vi "TankOverview.vi"() -> ()   [LabVIEW 2021]
uses:
  <vilib>/addons/control/pid/pid.llb/PID (DBL).vi
  <vilib>/addons/control/pid/NI_PID_pid.lvlib
panel:
  in  "Fout":dbl(slide) scale=0.0..10.0
  out "Tank":dbl(slide) scale=0.0..20.0
  out "Tank Level [cm]":dbl(graph)
  in  "PID gains":T1={"proportional gain (Kc)"=1.0, "integral time (Ti, min)"=0.01, "derivative time (Td, min)"=0.0} {"derivative time (Td, min)" format="%.3f"; "integral time (Ti, min)" format="%.3f"; "proportional gain (Kc)" format="%.3f"}
  in  "Hset":dbl(slide) scale=0.0..20.0
  in  "stop":bool
  in  "Ts [ms]":dbl
  in  "Tf [s]":dbl
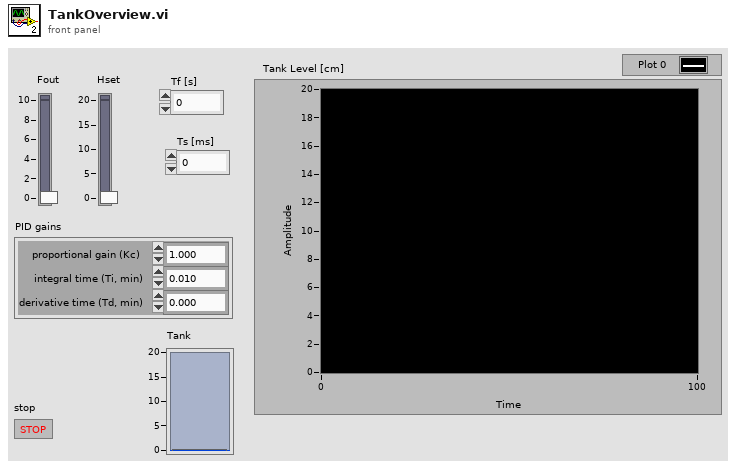
[diagram p1: front panel]
types:
  T1 = cluster{"proportional gain (Kc)":dbl, "integral time (Ti, min)":dbl, "derivative time (Td, min)":dbl}
  T2 = enum16{"Read", "Write", "ReadWrite", "BufferedRead", "BufferedReadWrite"}
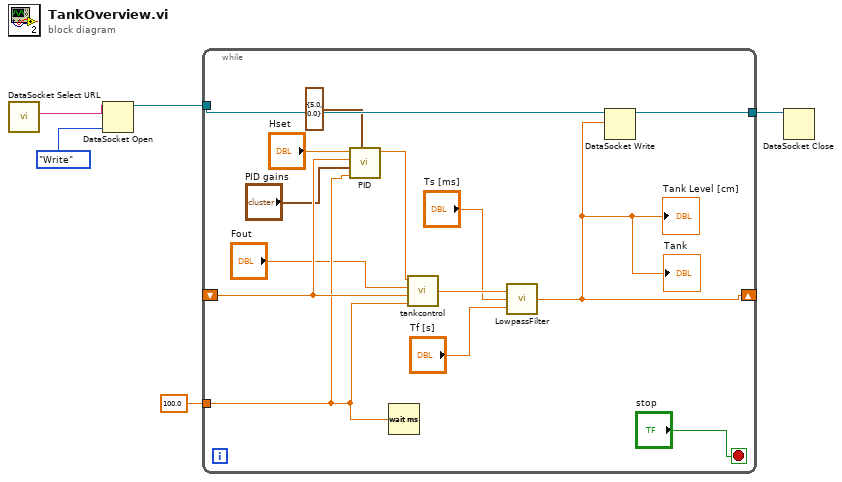
[diagram p0: block diagram]
diagram:
  n1 = call <vilib>:"DataSocket Select URL.vi"() -> ("URL"=w4:string)  [unwired: 9 in, 2 out]
  n2 = DataSocket Open(10:T2."Write" ("mode"), 11:w4) -> (3:w2:refnum<k13>)  [unwired: 2 in, 1 out]
  n3 = while {
    tunnel: 100.0 ("dt") -> [w9]
    shift-right: [w6] -> _
    shift-left: _ -> [w11]
    tunnel: w2 -> [w15]
    tunnel: [w14] -> w1
    stop <- "stop" stop-if-true
    n4 = call-poly <vilib>:"PID.vi"("output range"=cluster{"output high":dbl, "output low":dbl} {"output high"=5.0, "output low"=0.0}, "dt (s)"=w9, "PID gains"="PID gains", "process variable"=w11, "setpoint"="Hset") -> ("output"=w13:dbl)  [unwired: 5 in, 1 out]
    n5 = Wait (ms)(milliseconds to wait=w9) -> ()  [unwired: 1 out]
    n6 = call "tankcontrol.vi"("dt"=w9, "h(n)"=w11, "Fout [cm3/s]"="Fout", "U [V]"=w13) -> ("h(n+1)"=w19:dbl)
    n7 = call "LowpassFilter.vi"("Ts [ms]"="Ts [ms]", "Tf [s]"="Tf [s]", "Y(n)"=w19) -> ("Y(n+1)"=w6:dbl)
    "Tank Level [cm]" <- w6
    "Tank" <- w6
    n8 = DataSocket Write(10:w6, 11:w15) -> (3:w14:refnum<k13>)  [unwired: 2 in, 2 out]
  }
  n9 = DataSocket Close(11:w1) -> ()  [unwired: 2 in, 2 out]
